vi "MatrixSwitch.vi"(8 "error in (no error)":errorcluster, 10 "Action":T1(ring), 11 "LXIPXISwitching in":refnum<class "LXIPXISwitching.lvclass">) -> (0 "error out":errorcluster, 3 "LXIPXISwitching out":refnum<class "LXIPXISwitching.lvclass">)   [LabVIEW 2018, in "LXIPXISwitching.lvclass"]
uses:
  LXIPXISwitching.lvclass
  LXIPXISwitching.lvclass/LXIPXISwitching.ctl
  QCtests/general_VIs/globals/QC_MeasurementSetup.vi
panel:
  # "Pickering Matrix Settings"
  # "X1"
  # "X2"
  # "X3"
  # "X4"
  # "X5"
  # "X6"
  # "X7"
  # "X8"
  # "X9"
  # "X10"
  # "X11"
  # "X12"
  # "Y1"
  # "Y2"
  # "Y3"
  # "Y4"
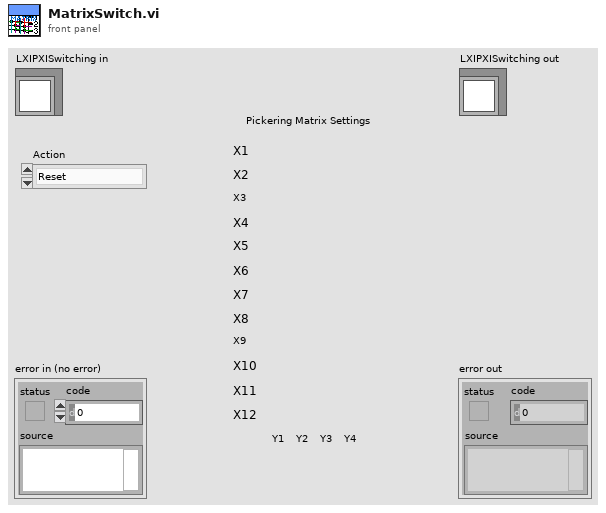
[diagram p1: front panel]
types:
  T1 = enum16{"Reset", "Ground", "Striptest SMU", "Striptest LCR", "IV", "CV", "Interstrip Cap", "Interstrip Res", "Setup StripTest"}
  T2 = cluster{"Supply":refnum<class "SupplyControl.lvclass">, "Initial Voltage [V]":dbl, "Final Voltage [V]":dbl, "Step Size [V]":dbl, "Step Interval [s]":i32, "Number Of Steps":u32, "Ramp down steps [V]":dbl, "Ramp down Interval [s]":i32, "Set Current Limit?":bool, "Current Limit [µA]":dbl, "Temperature Readout":enum16{"Read Arduino", "Enter manually"}, "Arduino":refnum<class "ArduinoControl.lvclass">, "Supply Name":string, "V_breakdown Limit [V]":dbl, "Switching":refnum<class "Switching.lvclass">}
  T3 = cluster{"Supply":refnum<class "SupplyControl.lvclass">, "LCR":refnum<class "LCRControl.lvclass">, "Initial Voltage [V]":dbl, "Final Voltage [V]":dbl, "Step Size [V]":dbl, "Step Interval [s]":i32, "Number Of Steps":u32, "AC frequency [Hz]":i32, "RC Configuration":u16, "AC amplitude [V]":dbl, "Ramp down steps [V]":dbl, "Ramp down Interval [s]":i32, "Set Current Limit?":bool, "Current Limit [µA]":dbl, "Temperature Readout":enum16{"Read Arduino", "Enter manually"}, "Arduino":refnum<class "ArduinoControl.lvclass">, "Supply Name":string, "LCR Name":string, "V_depletion Limit [V]":dbl, "Switching":refnum<class "Switching.lvclass">}
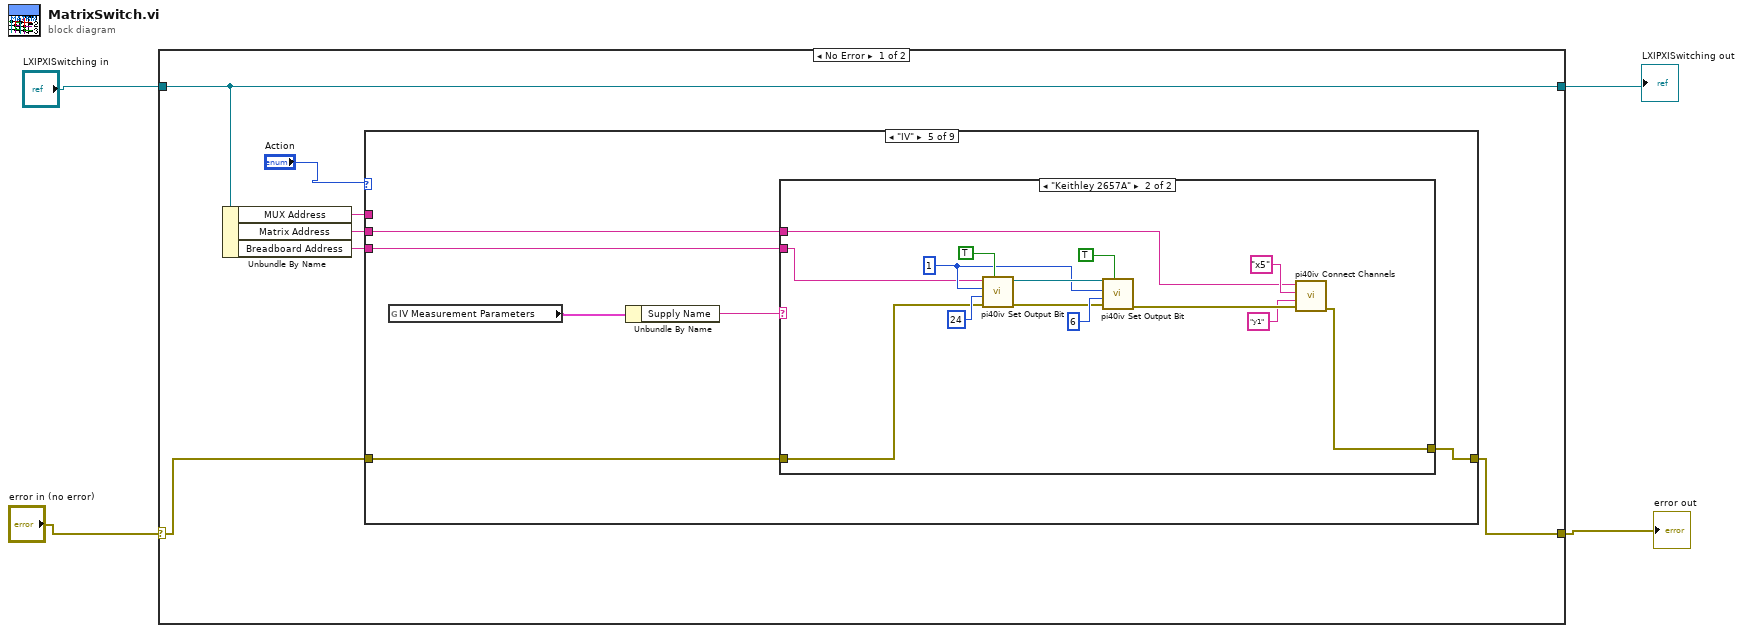
[diagram p0: block diagram]
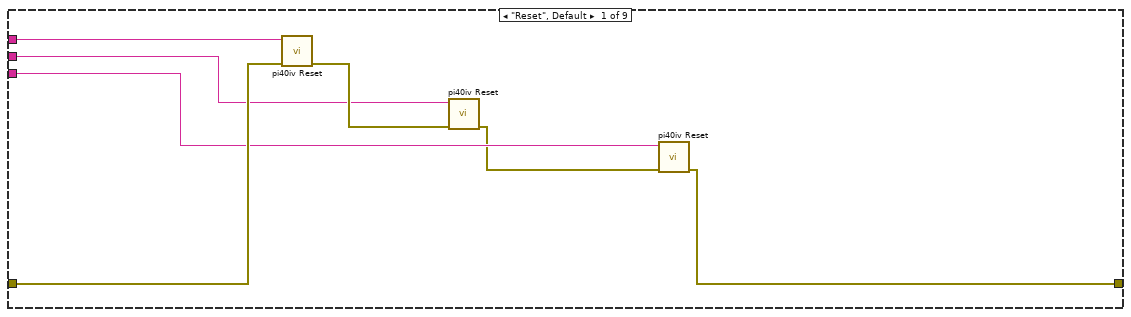
[diagram p2: hidden frame]
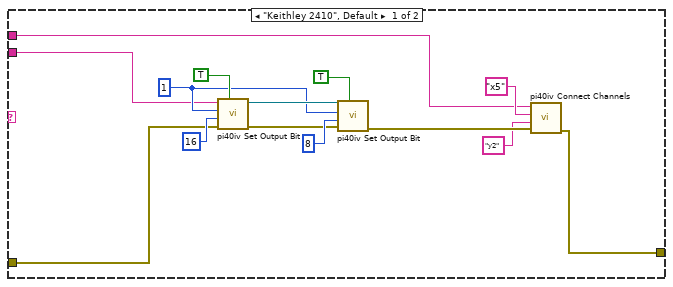
[diagram p6: hidden frame]
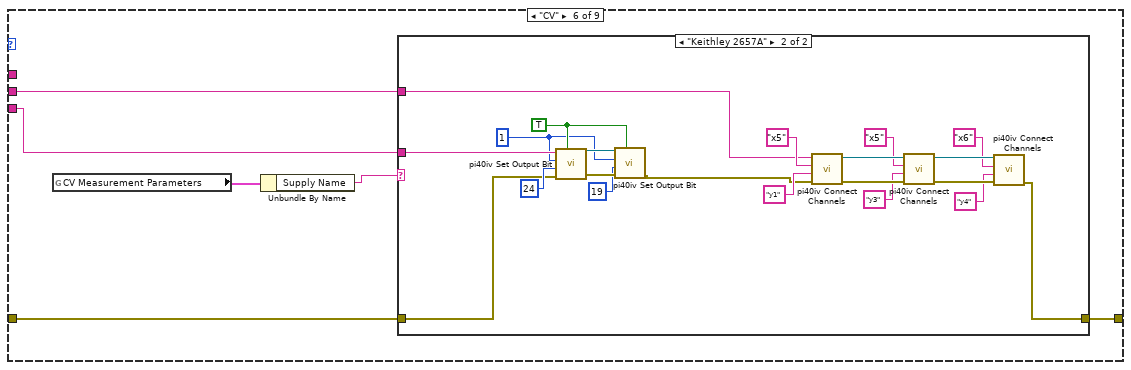
[diagram p7: hidden frame]
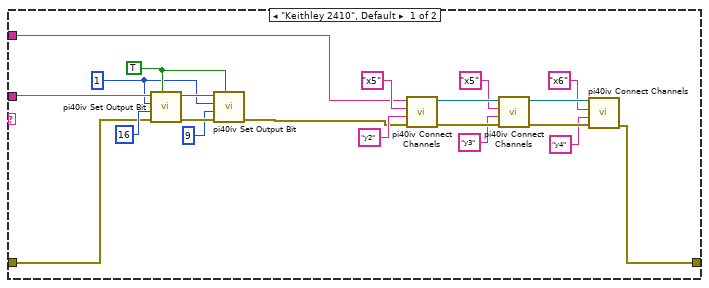
[diagram p8: hidden frame]
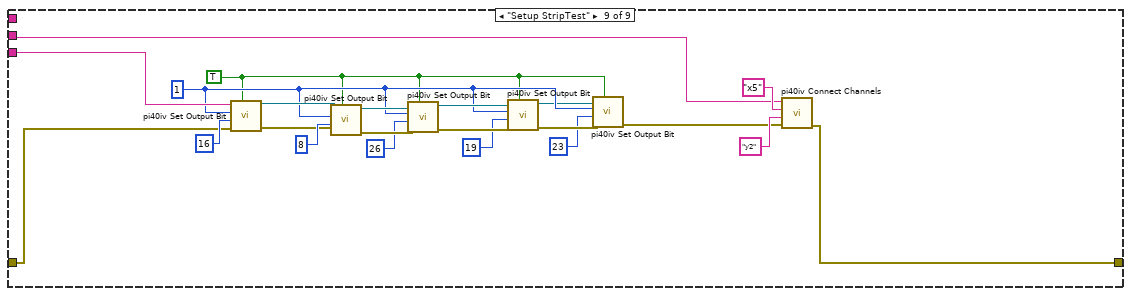
[diagram p11: hidden frame]
diagram:
  n1 = case shown="No Error" "error in (no error)" {
    selector: "error in (no error)" -> [w10 w128]
    tunnel: "LXIPXISwitching in" -> [w11 w129]
    tunnel: [w11 w129] -> w2
    tunnel: [w7 w128] -> w1
    frame No Error {
      n2 = Unbundle By Name(w11) -> ("MUX Address"=w6:string, "Matrix Address"=w8:string, "Breadboard Address"=w9:string)
      n3 = case shown="\"IV\"" "Action" {
        tunnel: w10 -> [w16 w19 w20 w21 w25 w58 w104 w105 w116]
        tunnel: w9 -> [w14 _ _ _ w24 w59 _ _ w121]
        tunnel: w8 -> [w15 _ _ _ w23 w57 _ _ w113]
        tunnel: [w12 w19 w20 w21 w22 w56 w104 w105 w107] -> w7
        tunnel: w6 -> [w17 _ _ _ _ _ _ _ _]
        frame "Reset", Default {
          n4 = call <instrlib>:"pi40iv Reset.vi"("error in (no error)"=w16, "instrument handle"=w17) -> ("error out"=w18:errorcluster)  [unwired: 8 in, 1 out]
          n5 = call <instrlib>:"pi40iv Reset.vi"("error in (no error)"=w18, "instrument handle"=w15) -> ("error out"=w13:errorcluster)  [unwired: 8 in, 1 out]
          n6 = call <instrlib>:"pi40iv Reset.vi"("error in (no error)"=w13, "instrument handle"=w14) -> ("error out"=w12:errorcluster)  [unwired: 8 in, 1 out]
        }
        frame "Ground" {
          # "To be implemented..."
        }
        frame "Striptest SMU" {
          # "To be Implemented..."
        }
        frame "Striptest LCR" {
          # "To be implemented..."
        }
        frame "IV" {
          n7 = global read "QC_MeasurementSetup.vi" "IV Measurement Parameters"() -> (w27:T2)
          n8 = Unbundle By Name(w27) -> ("Supply Name"=w26:string)
          n9 = case shown="\"Keithley 2657A\"" w26 {
            tunnel: w25 -> [w31 w43]
            tunnel: w24 -> [w30 w45]
            tunnel: w23 -> [w29 w44]
            tunnel: [w28 w42] -> w22
            frame "Keithley 2410", Default {
              w37 = u32 1 ("output sub number")
              n10 = call <instrlib>:"pi40iv Set Output Bit.vi"("state"=TRUE, "error in (no error)"=w31, "bit number"=u32 16, "output sub number"=w37, "instrument handle"=w30) -> ("error out"=w35:errorcluster, "instrument handle out"=w39:refnum<k15>)  [unwired: 5 in]
              n11 = call <instrlib>:"pi40iv Set Output Bit.vi"("state"=TRUE, "error in (no error)"=w35, "bit number"=u32 8, "output sub number"=w37, "instrument handle"=w39) -> ("error out"=w34:errorcluster)  [unwired: 5 in, 1 out]
              n12 = call <instrlib>:"pi40iv Connect Channels.vi"("error in (no error)"=w34, "channel 2"="y2", "channel 1"="x5", "instrument handle"=w29) -> ("error out"=w28:errorcluster)  [unwired: 6 in, 1 out]
            }
            frame "Keithley 2657A" {
              w51 = u32 1 ("output sub number")
              n13 = call <instrlib>:"pi40iv Set Output Bit.vi"("state"=TRUE, "error in (no error)"=w43, "bit number"=u32 24, "output sub number"=w51, "instrument handle"=w45) -> ("error out"=w49:errorcluster, "instrument handle out"=w53:refnum<k15>)  [unwired: 5 in]
              n14 = call <instrlib>:"pi40iv Set Output Bit.vi"("state"=TRUE, "error in (no error)"=w49, "bit number"=u32 6, "output sub number"=w51, "instrument handle"=w53) -> ("error out"=w48:errorcluster)  [unwired: 5 in, 1 out]
              n15 = call <instrlib>:"pi40iv Connect Channels.vi"("error in (no error)"=w48, "channel 2"="y1", "channel 1"="x5", "instrument handle"=w44) -> ("error out"=w42:errorcluster)  [unwired: 6 in, 1 out]
            }
          }
        }
        frame "CV" {
          n16 = global read "QC_MeasurementSetup.vi" "CV Measurement Parameters"() -> (w61:T3)
          n17 = Unbundle By Name(w61) -> ("Supply Name"=w60:string)
          n18 = case shown="\"Keithley 2657A\"" w60 {
            tunnel: w59 -> [w68 w89]
            tunnel: w58 -> [w67 w88]
            tunnel: w57 -> [w66 w87]
            tunnel: [w65 w86] -> w56
            frame "Keithley 2410", Default {
              w63 = u32 1 ("output sub number")
              w64 = TRUE ("state")
              n19 = call <instrlib>:"pi40iv Set Output Bit.vi"("state"=w64, "error in (no error)"=w67, "bit number"=u32 16, "output sub number"=w63, "instrument handle"=w68) -> ("error out"=w82:errorcluster, "instrument handle out"=w81:refnum<k15>)  [unwired: 5 in]
              n20 = call <instrlib>:"pi40iv Set Output Bit.vi"("state"=w64, "error in (no error)"=w82, "bit number"=u32 9, "output sub number"=w63, "instrument handle"=w81) -> ("error out"=w62:errorcluster)  [unwired: 5 in, 1 out]
              n21 = call <instrlib>:"pi40iv Connect Channels.vi"("error in (no error)"=w62, "channel 2"="y2", "channel 1"="x5", "instrument handle"=w66) -> ("error out"=w76:errorcluster, "instrument handle out"=w74:refnum<k15>)  [unwired: 6 in]
              n22 = call <instrlib>:"pi40iv Connect Channels.vi"("error in (no error)"=w76, "channel 2"="y3", "channel 1"="x5", "instrument handle"=w74) -> ("error out"=w75:errorcluster, "instrument handle out"=w73:refnum<k15>)  [unwired: 6 in]
              n23 = call <instrlib>:"pi40iv Connect Channels.vi"("error in (no error)"=w75, "channel 2"="y4", "channel 1"="x6", "instrument handle"=w73) -> ("error out"=w65:errorcluster)  [unwired: 6 in, 1 out]
            }
            frame "Keithley 2657A" {
              w84 = u32 1 ("output sub number")
              w85 = TRUE ("state")
              n24 = call <instrlib>:"pi40iv Set Output Bit.vi"("state"=w85, "error in (no error)"=w88, "bit number"=u32 24, "output sub number"=w84, "instrument handle"=w89) -> ("error out"=w103:errorcluster, "instrument handle out"=w102:refnum<k15>)  [unwired: 5 in]
              n25 = call <instrlib>:"pi40iv Set Output Bit.vi"("state"=w85, "error in (no error)"=w103, "bit number"=u32 19, "output sub number"=w84, "instrument handle"=w102) -> ("error out"=w83:errorcluster)  [unwired: 5 in, 1 out]
              n26 = call <instrlib>:"pi40iv Connect Channels.vi"("error in (no error)"=w83, "channel 2"="y1", "channel 1"="x5", "instrument handle"=w87) -> ("error out"=w97:errorcluster, "instrument handle out"=w95:refnum<k15>)  [unwired: 6 in]
              n27 = call <instrlib>:"pi40iv Connect Channels.vi"("error in (no error)"=w97, "channel 2"="y3", "channel 1"="x5", "instrument handle"=w95) -> ("error out"=w96:errorcluster, "instrument handle out"=w94:refnum<k15>)  [unwired: 6 in]
              n28 = call <instrlib>:"pi40iv Connect Channels.vi"("error in (no error)"=w96, "channel 2"="y4", "channel 1"="x6", "instrument handle"=w94) -> ("error out"=w86:errorcluster)  [unwired: 6 in, 1 out]
            }
          }
        }
        frame "Interstrip Cap" {
          # "Needs to be integrated..."
        }
        frame "Interstrip Res" {
          # "Needs to be integrated..."
        }
        frame "Setup StripTest" {
          w111 = u32 1 ("output sub number")
          w110 = TRUE ("state")
          n29 = call <instrlib>:"pi40iv Set Output Bit.vi"("state"=w110, "error in (no error)"=w116, "bit number"=u32 16, "output sub number"=w111, "instrument handle"=w121) -> ("error out"=w124:errorcluster, "instrument handle out"=w126:refnum<k15>)  [unwired: 5 in]
          n30 = call <instrlib>:"pi40iv Set Output Bit.vi"("state"=w110, "error in (no error)"=w124, "bit number"=u32 8, "output sub number"=w111, "instrument handle"=w126) -> ("error out"=w118:errorcluster, "instrument handle out"=w120:refnum<k15>)  [unwired: 5 in]
          n31 = call <instrlib>:"pi40iv Set Output Bit.vi"("state"=w110, "error in (no error)"=w118, "bit number"=u32 26, "output sub number"=w111, "instrument handle"=w120) -> ("error out"=w117:errorcluster, "instrument handle out"=w119:refnum<k15>)  [unwired: 5 in]
          n32 = call <instrlib>:"pi40iv Set Output Bit.vi"("state"=w110, "error in (no error)"=w117, "bit number"=u32 19, "output sub number"=w111, "instrument handle"=w119) -> ("error out"=w112:errorcluster, "instrument handle out"=w106:refnum<k15>)  [unwired: 5 in]
          n33 = call <instrlib>:"pi40iv Set Output Bit.vi"("state"=w110, "error in (no error)"=w112, "bit number"=u32 23, "output sub number"=w111, "instrument handle"=w106) -> ("error out"=w108:errorcluster)  [unwired: 5 in, 1 out]
          n34 = call <instrlib>:"pi40iv Connect Channels.vi"("error in (no error)"=w108, "channel 2"="y2", "channel 1"="x5", "instrument handle"=w113) -> ("error out"=w107:errorcluster)  [unwired: 6 in, 1 out]
        }
      }
    }
    frame Error {
    }
  }
  "error out" <- w1
  "LXIPXISwitching out" <- w2
